vi "HoppingStep(NoZFeedback).vi"() -> ()   [LabVIEW 2014]
uses:
  <vilib>/Platform/TimedLoop/XDataNode/timing_clust.ctl
  <vilib>/Platform/TimedLoop/XDataNode/nitl_modes.ctl
  <vilib>/Platform/TimedLoop/XDataNode/wakeup.ctl
  <vilib>/rvi/Emulation/niFpgaGetClockAttributes.vi
  <vilib>/rvi/Emulation/niFpgaSctlEmulationGetInTimedLoop.vi
  <vilib>/rvi/Emulation/niFpgaEmulationReportErrorSimple.vi
  <vilib>/rvi/eio/common/nirviEmuTemplateMethod_errors.vi
  <vilib>/rvi/Emulation/niFpgaCriticalErrorInLSC.vi
  <vilib>/rvi/interface/RandomDataEmulation/niFpgaRandomDataHandleErrors.vi
  <vilib>/eio/EIONode/EIONode.xnode
  <vilib>/Platform/TimedLoop/XDataNode/XDataNode.xnode
  <vilib>/rvi/DataTransferAndStorage/Container/XNode/niFpgaContainer.xnode
  <vilib>/rvi/interface/RandomDataEmulation/nirviRandomDataFpgaReadWriteTemplate.vi
  <vilib>/Platform/TimedLoop/XDataNode/XDNodeRunTimeDep.lvlib
panel:
  out "XNum 2":i16
  out "Z":i16(graph)
  out "Waveform Chart":i16(graph)
  in  "stop":bool
  in  "ZOffset":i16
  in  "XOffset":i16
  in  "XNum":i16
  in  "XStepIndex":i16
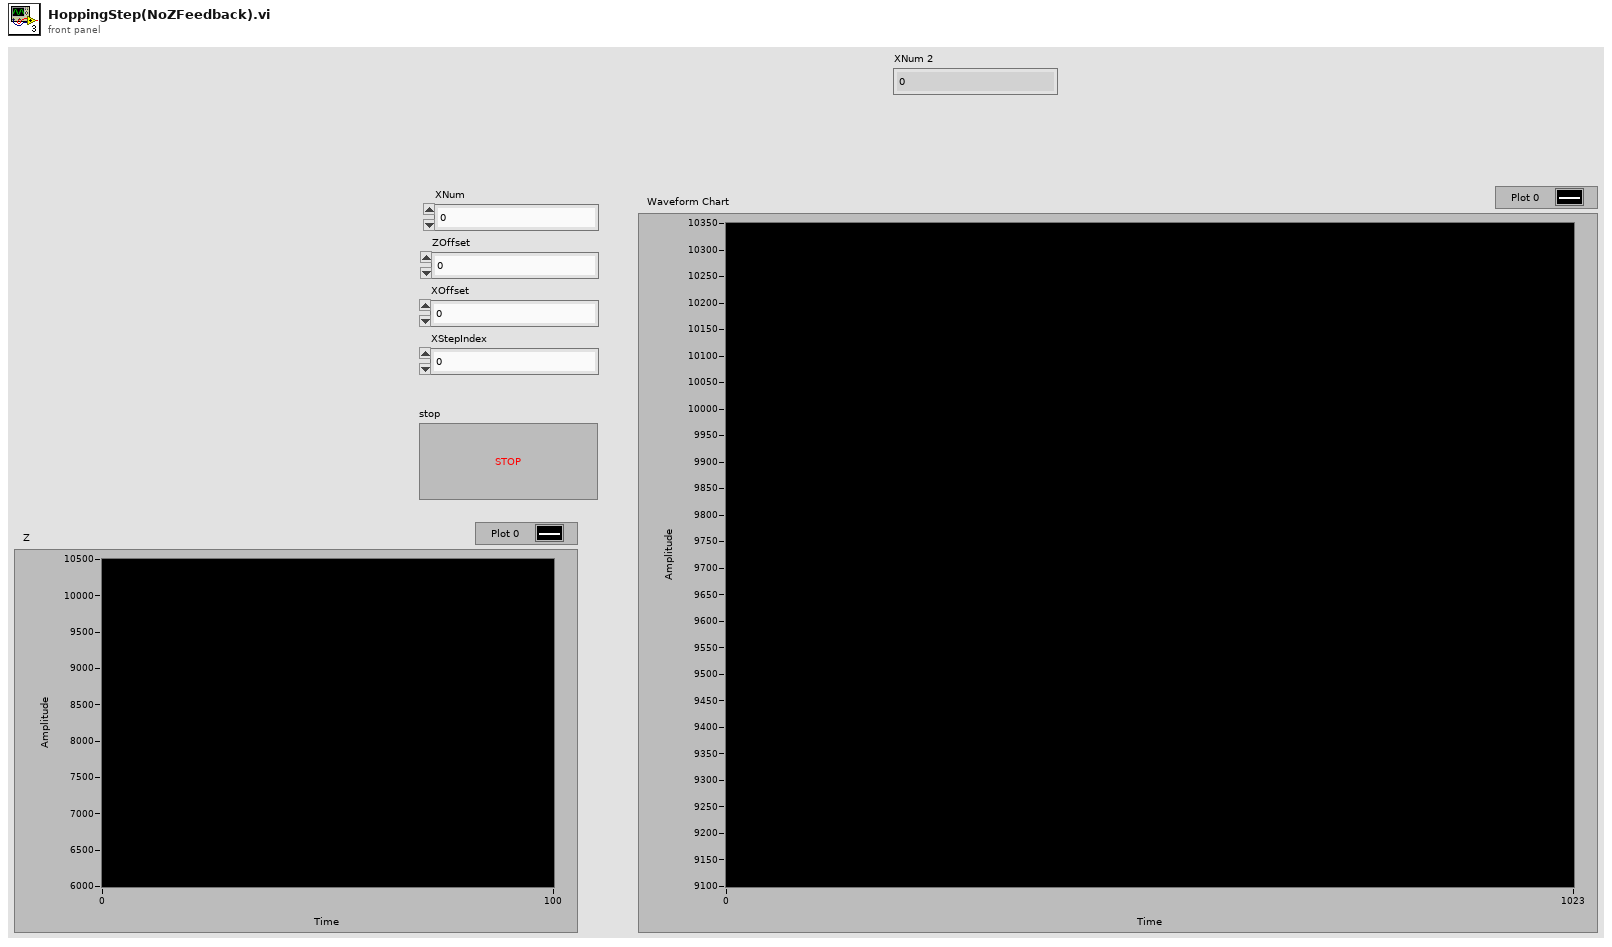
[diagram p1: front panel]
types:
  T1 = typedef "XDNodeRunTimeDep.lvlib/timing_clust.ctl" = cluster{"Expected End [f-1]":u64, "Actual End [f-1]":u64, "Finished Late? [f-1]":bool, "Expected End [i-1]":u64, "Actual End [i-1]":u64, "Finished Late? [i-1]":bool, "Expected Start [i]":u64, "Actual Start [i]":u64, "Expected Start [f]":u64, "Actual Start [f]":u64, "Source Name":string, "Structure Name":string, "Period":i64, "Deadline":i64, "Offset":i64, "Start":i64, "Priority":i32, "Timeout":i32, "Mode":T2, "Wakeup Reason":T3, "Error":errorcluster, "Source Type":string, "Secondary Source Type":string, "Global End Time":u64, "Global Start Time":u64, "Frame Duration":u64, "Iteration Duration":u64, "Assigned CPU":i32, "I/O Scan Engine Mode":u32}
  T2 = typedef "XDNodeRunTimeDep.lvlib/nitl_modes.ctl" = enum32{"No Change", "Process missed periods, maintain original phase", "Discard missed periods, maintain original phase", "Process missed periods, ignore original phase", "Discard missed periods, ignore original phase"}
  T3 = typedef "XDNodeRunTimeDep.lvlib/wakeup.ctl" = enum32{"Normal", "Aborted", "Asynchronous wakeup", "Timing source error", "Timed loop error", "Timeout"}
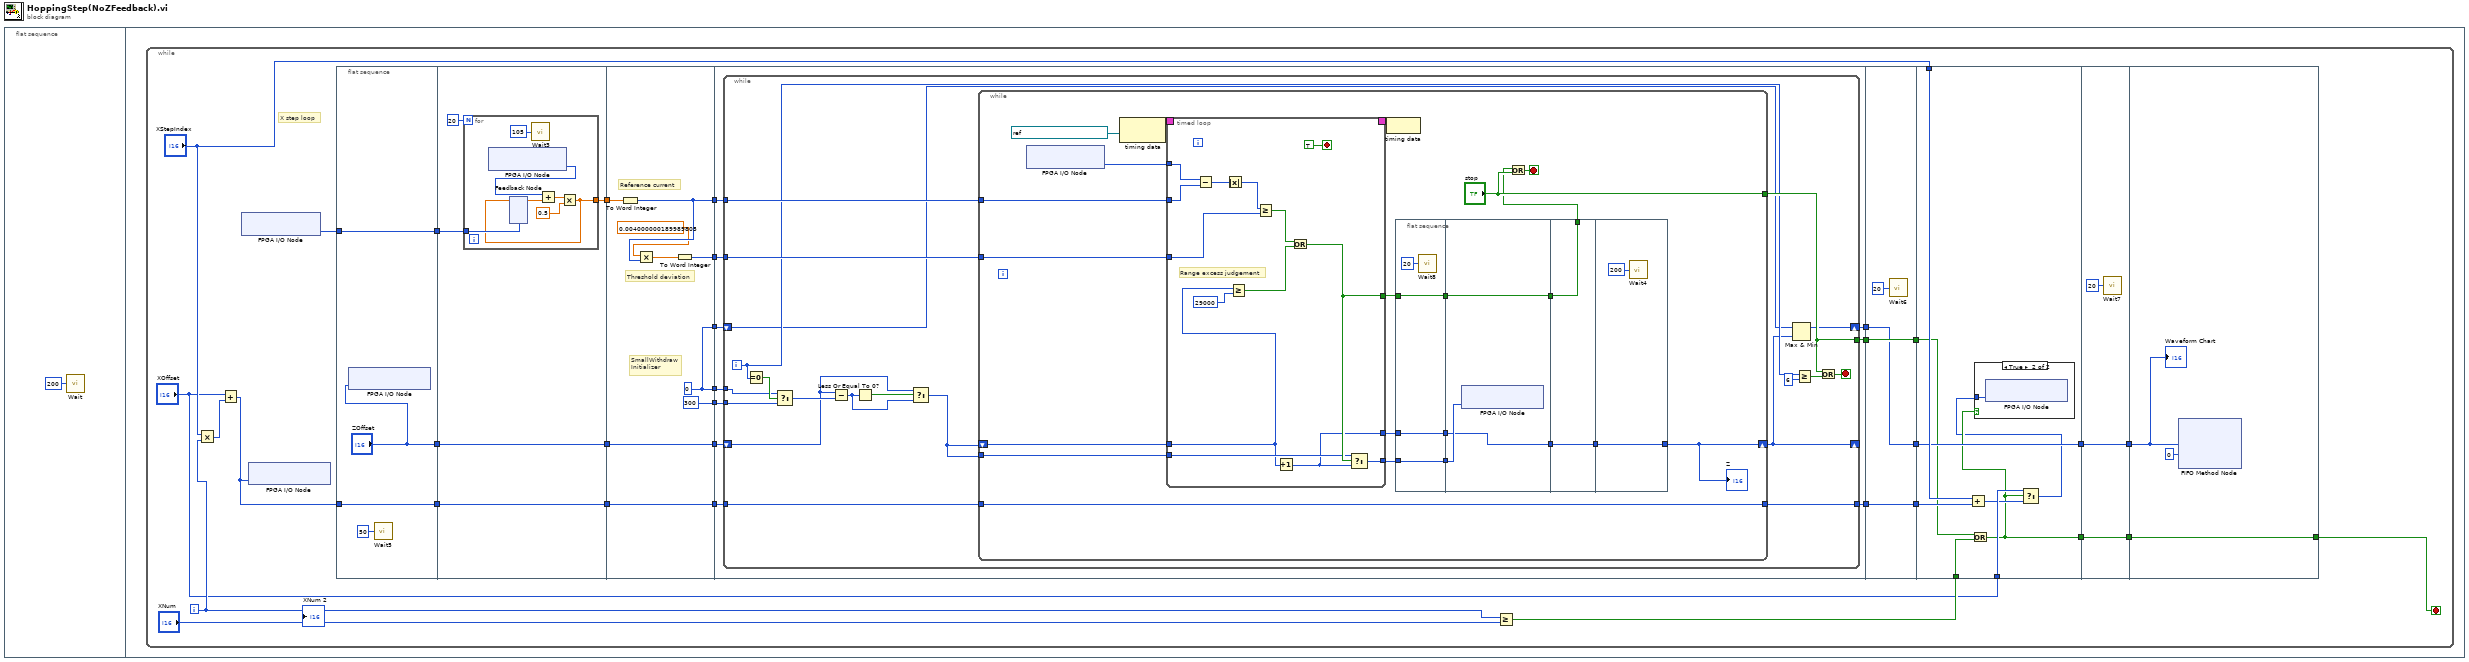
[diagram p0: block diagram]
diagram:
  n1 = flat-sequence {
    frame #0 {
      n2 = call "Wait"("Count(mSec)"=u32 200 ("Count(uSec)")) -> ()  [unwired: 1 out]
    }
    frame #1 {
      n3 = while {
        i -> [w8]
        stop <- w14 stop-if-true
        # "X step loop"
        n4 = Multiply(x="XStepIndex", y=w8) -> (x*y=w6:i32)
        n5 = Add(x="XOffset", y=w6) -> (x+y=w9:i32)
        n6 = xnode "FPGA I/O Node"() -> ("Connector0/AI1"=w22:i16)  [unwired: 1 in, 1 out]
        n7 = xnode "FPGA I/O Node"("Connector0/AO2"=w9) -> ()  [unwired: 1 in, 1 out]
        n8 = flat-sequence {
          tunnel: [w37] -> w31
          tunnel: [w35] -> w29
          tunnel: w9 -> [w37]
          tunnel: w22 -> [w35]
          tunnel: ["ZOffset"] -> w11
          tunnel: w31 -> [w42]
          tunnel: [w42] -> w32
          tunnel: w29 -> [w41]
          tunnel: [w39] -> w28
          tunnel: [w38] -> w12
          tunnel: w11 -> [w38]
          tunnel: [w51] -> w33
          tunnel: w32 -> [w58]
          tunnel: [w58] -> w30
          tunnel: w28 -> [w57]
          tunnel: [w56] -> w27
          tunnel: [w53] -> w26
          tunnel: [i16 300] -> w13
          tunnel: w12 -> [w51]
          tunnel: [w50] -> w4
          tunnel: [w50] -> w3
          tunnel: w26 -> [w65]
          tunnel: w27 -> [w66]
          tunnel: w30 -> [w68]
          tunnel: w33 -> [w67]
          tunnel: [w64] -> w23
          tunnel: [w63] -> w18
          tunnel: w13 -> [w62]
          tunnel: w4 -> [w61]
          tunnel: w3 -> [w60]
          tunnel: [w59] -> w2
          tunnel: [w142] -> w25
          tunnel: [w144] -> w24
          tunnel: w23 -> [w144]
          tunnel: [w143] -> w19
          tunnel: w18 -> [w143]
          tunnel: w2 -> [w142]
          tunnel: "XStepIndex" -> [w153]
          tunnel: w25 -> [w152]
          tunnel: w24 -> [w154]
          tunnel: [w152] -> w21
          tunnel: w19 -> [w151]
          tunnel: w17 -> [w150]
          tunnel: "XOffset" -> [w149]
          tunnel: [w147] -> w15
          tunnel: w21 -> [w157]
          tunnel: [w157] -> w20
          tunnel: [w156] -> w16
          tunnel: w15 -> [w156]
          tunnel: w20 -> [w159]
          tunnel: [w160] -> w14
          tunnel: w16 -> [w160]
          frame #0 {
            n9 = xnode "FPGA I/O Node"("Connector0/AO0"="ZOffset") -> ()  [unwired: 1 in, 1 out]
            n10 = call "Wait5"("Count(uSec)"=u32 50) -> ()  [unwired: 1 out]
          }
          frame #1 {
            n11 = for {
              N: 20 -> [_]
              tunnel: w41 -> [w48]
              tunnel: [w43] -> w39
              n12 = xnode "FPGA I/O Node"() -> ("Connector0/AI1"=w46:i16)  [unwired: 1 in, 1 out]
              n13 = feedback #1(w48) -> (w47:sgl)
              n14 = call "Wait3"("Count(uSec)"=u32 105) -> ()  [unwired: 1 out]
              n15 = Add(x=w46, y=w47) -> (x+y=w45:sgl)
              n16 = Multiply(x=w45, y=sgl 0.5) -> (x*y=w43:sgl)
              n17 = feedback-in #1(w43) -> ()
            }
          }
          frame #2 {
            w50 = i16 0
            # "SmallWithdraw\nInitializer"
            # "Threshold deviation"
            # "Reference current"
            n18 = To Word Integer(number=w57) -> (16bit integer=w56:i16)
            n19 = Multiply(x=sgl 0.004, y=w56) -> (x*y=w54:sgl)
            n20 = To Word Integer(number=w54) -> (16bit integer=w53:i16)
          }
          frame #3 {
            n21 = while {
              tunnel: w68 -> [w88]
              tunnel: w66 -> [w87]
              tunnel: w65 -> [w86]
              tunnel: [w84] -> w64
              tunnel: [w81] -> w63
              tunnel: w62 -> [w78]
              shift-right: [w70] -> _
              shift-left: w67 -> [w75]
              tunnel: w61 -> [w72]
              shift-right: [w69] -> w59
              shift-left: w60 -> [w71]
              i -> [w80]
              stop <- w83 stop-if-true
              n22 = Equal To 0?(x=w80) -> (x = 0?=w79:bool)
              n23 = Select(t=w72, s=w79, f=w78) -> (s? t:f=w77:i16)
              n24 = Subtract(x=w75, y=w77) -> (x-y=w74:i16)
              n25 = Less Or Equal To 0?(x=w74) -> (x <= 0?=w76:bool)
              n26 = Select(t=w75, s=w76, f=w74) -> (s? t:f=w73:i16)
              n27 = while {
                tunnel: w88 -> [w107]
                tunnel: w87 -> [w102]
                tunnel: w86 -> [w104]
                tunnel: [w107] -> w84
                tunnel: ["stop"] -> w81
                shift-right: [w93] -> w70
                shift-left: w73 -> [w99]
                tunnel: w73 -> [w96]
                stop <- w106 stop-if-true
                n28 = xnode "FPGA I/O Node"() -> ("Connector0/AI1"=w103:i16)  [unwired: 1 in, 1 out]
                n29 = node-c288(refnum<k21> "40 MHz Onboard Clock" ("Source Name")) -> (w110:T1)
                n30 = timed-loop {
                  timing: w110 -> [_]
                  timing-out: [_] -> w109
                  tunnel: w102 -> [w133]
                  tunnel: w104 -> [w130]
                  tunnel: w103 -> [w134]
                  tunnel: [w127] -> w100
                  tunnel: [w126] -> w98
                  tunnel: w99 -> [w124]
                  tunnel: w96 -> [w125]
                  tunnel: [w123] -> w95
                  stop <- TRUE stop-if-true
                  # "Range excess judgement"
                  n31 = Subtract(x=w134, y=w133) -> (x-y=w132:i16)
                  n32 = Absolute Value(x=w132) -> (abs(x)=w131:i16)
                  n33 = Greater Or Equal?(x=w124, y=i16 29000) -> (x >= y?=w128:bool)
                  n34 = Greater Or Equal?(x=w131, y=w130) -> (x >= y?=w129:bool)
                  n35 = Increment(x=w124) -> (x+1=w123:i16)
                  n36 = Or(x=w129, y=w128) -> (x .or. y?=w126:bool)
                  n37 = Select(t=w125, s=w126, f=w123) -> (s? t:f=w127:i16)
                }
                n38 = node-c288(w109) -> ()
                n39 = flat-sequence {
                  tunnel: [w113] -> w101
                  tunnel: w100 -> [w113]
                  tunnel: w98 -> [w112]
                  tunnel: [w112] -> w97
                  tunnel: w95 -> [w111]
                  tunnel: [w111] -> w94
                  tunnel: w101 -> [w117]
                  tunnel: [w116] -> w92
                  tunnel: w97 -> [w115]
                  tunnel: w94 -> [w116]
                  tunnel: [w115] -> w90
                  tunnel: w92 -> [w119]
                  tunnel: [w119] -> w91
                  tunnel: w90 -> [w118]
                  tunnel: [w118] -> w89
                  tunnel: w91 -> [w120]
                  tunnel: [w120] -> w93
                  frame #0 {
                    n40 = call "Wait8"("Count(uSec)"=u32 20) -> ()  [unwired: 1 out]
                  }
                  frame #1 {
                    n41 = xnode "FPGA I/O Node"("Connector0/AO0"=w117) -> ()  [unwired: 1 in, 1 out]
                  }
                  frame #2 {
                  }
                  frame #3 {
                    n42 = call "Wait4"("Count(uSec)"=u32 200) -> ()  [unwired: 1 out]
                  }
                }
                n43 = Or(x=w89, y="stop") -> (x .or. y?=w106:bool)
                "Z" <- w93
              }
              n44 = Max & Min(x=w71, y=w70) -> (max(x,y)=w69:i16)  [unwired: 1 out]
              n45 = Greater Or Equal?(x=w80, y=6) -> (x >= y?=w82:bool)
              n46 = Or(x=w81, y=w82) -> (x .or. y?=w83:bool)
            }
          }
          frame #4 {
            n47 = call "Wait6"("Count(uSec)"=u32 20) -> ()  [unwired: 1 out]
          }
          frame #5 {
            n48 = Add(x=w153, y=w154) -> (x+y=w148:i32)
            n49 = Or(x=w151, y=w150) -> (x .or. y?=w147:bool)
            n50 = Select(t=w149, s=w147, f=w148) -> (s? t:f=w146:i32)
            n51 = case shown="True" w147 {
              tunnel: w146 -> [_ w155]
              frame False {
              }
              frame True {
                n52 = xnode "FPGA I/O Node"("Connector0/AO2"=w155) -> ()  [unwired: 1 in, 1 out]
              }
            }
          }
          frame #6 {
            n53 = call "Wait7"("Count(uSec)"=u32 20) -> ()  [unwired: 1 out]
          }
          frame #7 {
            n54 = xnode ("FIFO Method Node")("Element"=w159, "Timeout"=0) -> ()  [unwired: 1 in, 2 out]
            "Waveform Chart" <- w159
          }
        }
        n55 = Greater Or Equal?(x=w8, y="XNum") -> (x >= y?=w17:bool)
        "XNum 2" <- "XNum"
      }
    }
  }
